vi "Contains.vi"(8 "error in (no error)":errorcluster, 9 "Item":refnum<class "ILabVIEWItem.lvclass">, 11 "CLabVIEWContainer in":refnum<class "CLabVIEWContainer.lvclass">) -> (0 "error out":errorcluster, 2 "Contains?":bool, 3 "CLabVIEWContainer out":refnum<class "CLabVIEWContainer.lvclass">)   [LabVIEW 2020, in "LabVIEWContainers.lvlib" / "CLabVIEWContainer.lvclass"]
uses:
  CLabVIEWContainer.lvclass
  obj/Addons/LabVIEWObjectInterfaces.lvlibp/LabVIEWObjectInterfaces/ILabVIEWItem/ILabVIEWItem.lvclass
  CLabVIEWContainer.lvclass/CLabVIEWContainer.ctl
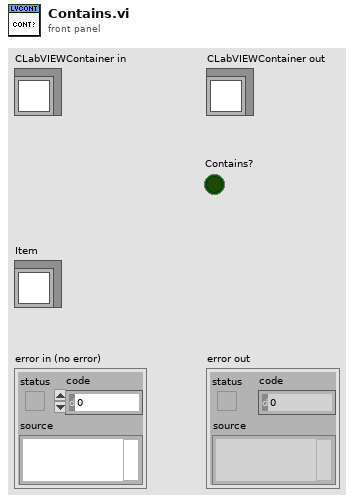
[diagram p1: front panel]
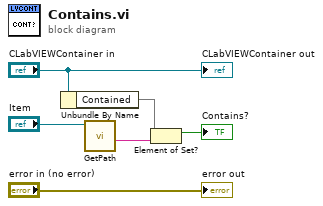
[diagram p0: block diagram]
diagram:
  n1 = Unbundle By Name("CLabVIEWContainer in") -> ("Contained"=w5:set{string})
  n2 = call-dynamic "GetPath.vi"("ILabVIEWItem in"="Item") -> ("Path"=w1:string)  [unwired: 8 in, 2 out]
  n3 = Element of Set?(10:w1, 11:w5) -> (3:→"Contains?":bool)
  "error out" <- "error in (no error)"
  "CLabVIEWContainer out" <- "CLabVIEWContainer in"
